vi "Create (Cluster).vi"(7 "Options":T1, 8 "error in (no error)":errorcluster, 10 "Base URL (None)":string, 11 "URL Pattern Init":T2) -> (0 "error out":errorcluster, 3 "URLPattern out":refnum<class "URLPattern.lvclass">)   [LabVIEW 2020, in "Stream.lvlib" / "URLPattern.lvclass"]
uses:
  URLPattern.lvclass
  URL Pattern Init.ctl
  Options.ctl
  URLPattern.lvclass/URLPattern.ctl
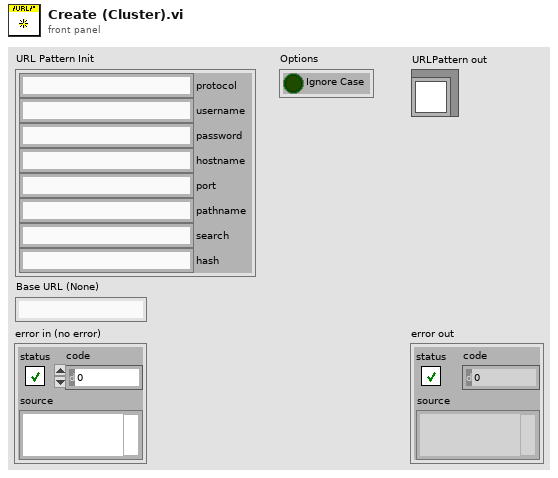
[diagram p1: front panel]
types:
  T1 = typedef "Stream.lvlib/URLPattern.lvclass/Options.ctl" = cluster{"Ignore Case":bool}
  T2 = typedef "Stream.lvlib/URLPattern.lvclass/URL Pattern Init.ctl" = cluster{"protocol":string, "username":string, "password":string, "hostname":string, "port":string, "pathname":string, "search":string, "hash":string}
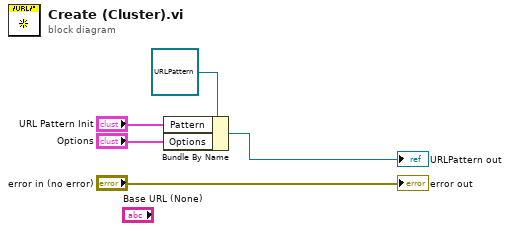
[diagram p0: block diagram]
diagram:
  n1 = Bundle By Name(cluster=refnum<class "URLPattern.lvclass"> refnum ("URLPattern in"), "Pattern"="URL Pattern Init", "Options"="Options") -> (→"URLPattern out":refnum<class "URLPattern.lvclass">)
  "error out" <- "error in (no error)"
